vi "mkROIsToString.vi"(11 "Settings":T1={"Gain [1-4]"=1.0, "Offset"=50, "Mode"=6, "ROIs"=[], "ROI Size"={"X"=0, "Y"=0}, "Number of buffers"=40, "Use hardware multiple-ROI?"=TRUE, "GenericCameraConfig"={"Framerate (Hz)"=60, "Exposure time (us)"=5000, "Image size"={"Width"=1280, "Height"=1024}}} {"Offset" min=50}) -> (3 "ROIs description":string)   [LabVIEW 2011]
uses:
  CameraConfig.ctl
  BeadTracker2.llb/GenericCameraConfigType.ctl
panel:
  # "us"
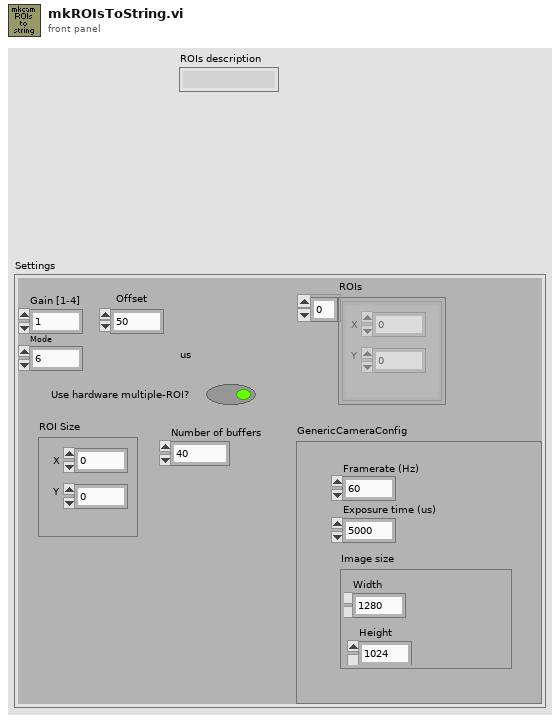
[diagram p1: front panel]
types:
  T1 = typedef "CameraConfig.ctl" = cluster{"Gain [1-4]":sgl, "Offset":i16, "Mode":i16, "ROIs":cluster{"X":i32, "Y":i32}[], "ROI Size":cluster{"X":i32, "Y":i32}, "Number of buffers":i32, "Use hardware multiple-ROI?":bool, "GenericCameraConfig":T2}
  T2 = typedef "GenericCameraConfigType.ctl" = cluster{"Framerate (Hz)":i32, "Exposure time (us)":i32, "Image size":cluster{"Width":i32, "Height":i32}}
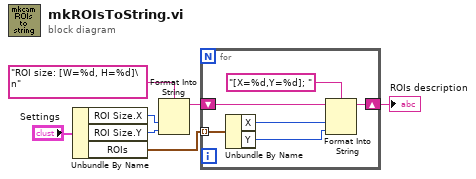
[diagram p0: block diagram]
diagram:
  n1 = Unbundle By Name("Settings") -> ("ROI Size.X"=w4:i32, "ROI Size.Y"=w3:i32, "ROIs"=w6:cluster{"X":i32, "Y":i32}[])
  n2 = Format Into String(format string="ROI size: [W=%d, H=%d]\n", w4, w3) -> (resulting string=w2:string)  [unwired: 2 in, 1 out]
  n3 = for {
    tunnel: w6 -> [w11] mode=indexing
    shift-right: [w8] -> w1
    shift-left: w2 -> [w13]
    n4 = Unbundle By Name(w11) -> ("X"=w10:i32, "Y"=w9:i32)
    n5 = Format Into String(format string="[X=%d,Y=%d]; ", initial string=w13, w10, w9) -> (resulting string=w8:string)  [unwired: 1 in, 1 out]
  }
  "ROIs description" <- w1
